vi "FPGA_ZAdjustment.vi"() -> ()   [LabVIEW 2014]
uses:
  <vilib>/rvi/Emulation/niFpgaGetClockAttributes.vi
  <vilib>/rvi/Emulation/niFpgaSctlEmulationGetInTimedLoop.vi
  <vilib>/rvi/Emulation/niFpgaEmulationReportErrorSimple.vi
  <vilib>/rvi/eio/common/nirviEmuTemplateMethod_errors.vi
  <vilib>/rvi/Emulation/niFpgaCriticalErrorInLSC.vi
  <vilib>/rvi/Emulation/niFpgaProcessEmulError.vi
  <vilib>/rvi/interface/RandomDataEmulation/niFpgaRandomDataHandleErrors.vi
  <vilib>/eio/EIONode/EIONode.xnode
  <vilib>/rvi/DataTransferAndStorage/Container/XNode/niFpgaContainer.xnode
  <vilib>/rvi/interface/RandomDataEmulation/nirviRandomDataFpgaReadWriteTemplate.vi
panel:
  out "Connector0/DIO0":bool
  out "Connector0/DIO1":bool
  out "Connector0/DIO2":bool
  out "ZRealTimePos":i16
  in  "stop":bool
  in  "ZOffset":i16
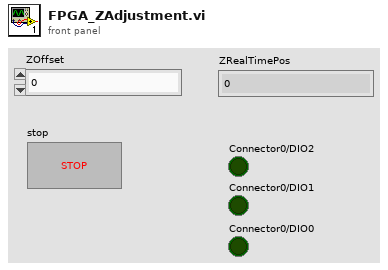
[diagram p1: front panel]
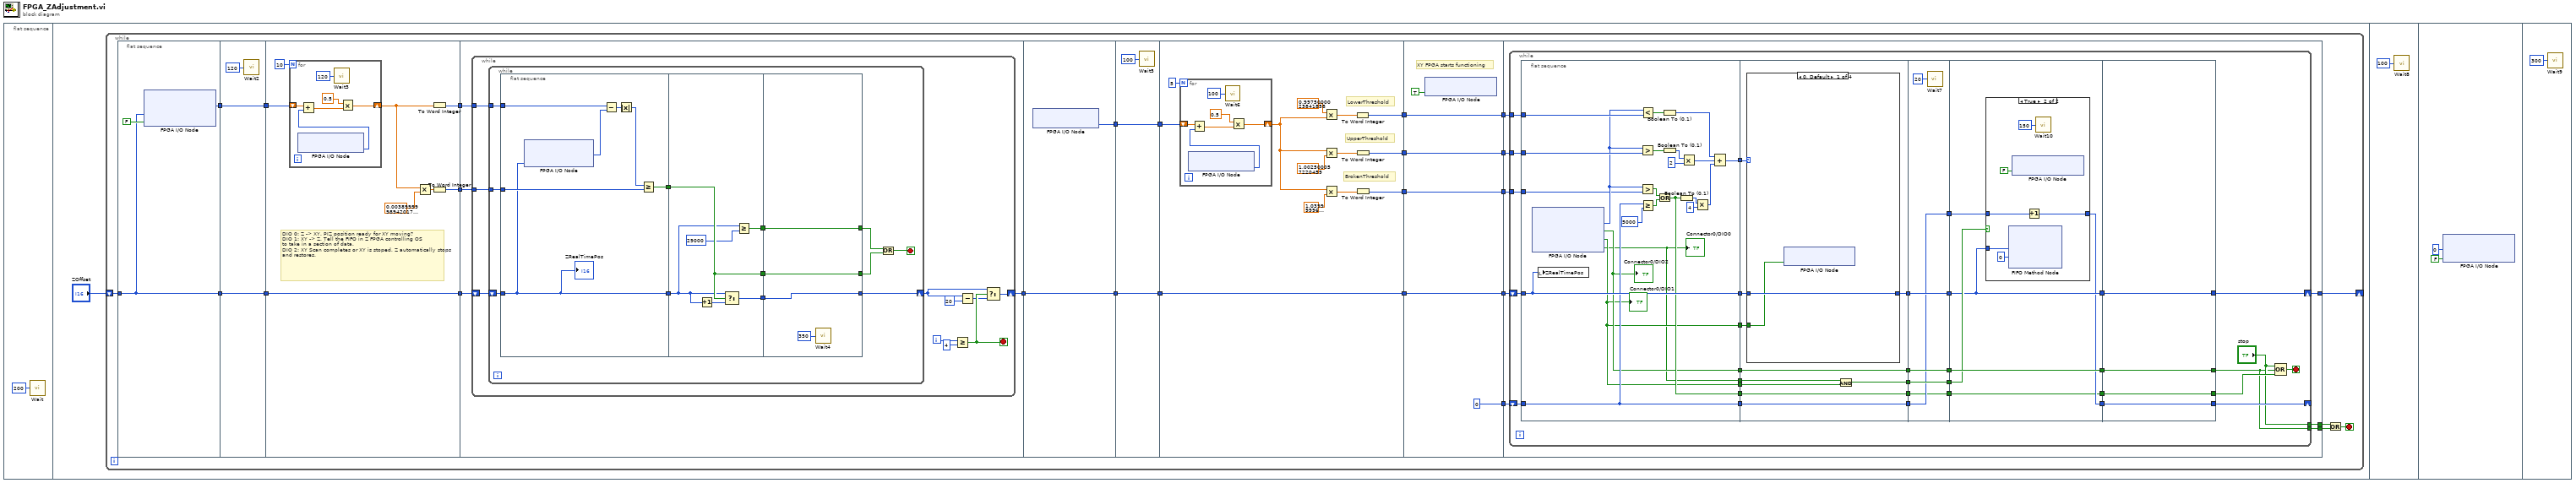
[diagram p0: block diagram]
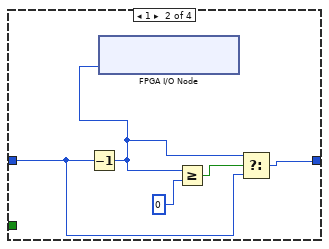
[diagram p2: hidden frame]
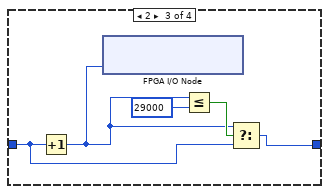
[diagram p3: hidden frame]
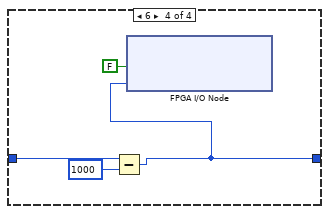
[diagram p4: hidden frame]
diagram:
  n1 = flat-sequence {
    frame #0 {
      n2 = call "Wait"("Count(uSec)"=u32 200) -> ()  [unwired: 1 out]
    }
    frame #1 {
      n3 = while {
        shift-right: [w7] -> _
        shift-left: "ZOffset" -> [w24]
        stop <- w5 stop-if-true
        n4 = flat-sequence {
          tunnel: [w31] -> w27
          tunnel: w24 -> [w29]
          tunnel: [w29] -> w22
          tunnel: [w33] -> w28
          tunnel: w27 -> [w33]
          tunnel: [w32] -> w23
          tunnel: w22 -> [w32]
          tunnel: w28 -> [w41]
          tunnel: [w37] -> w26
          tunnel: [w36] -> w25
          tunnel: w23 -> [w35]
          tunnel: [w35] -> w21
          tunnel: w26 -> [w52]
          tunnel: w25 -> [w51]
          tunnel: w21 -> [w50]
          tunnel: [w49] -> w20
          tunnel: w20 -> [w92]
          tunnel: [w93] -> w19
          tunnel: [w92] -> w10
          tunnel: w19 -> [w95]
          tunnel: [w95] -> w18
          tunnel: [w94] -> w11
          tunnel: w10 -> [w94]
          tunnel: w18 -> [w108]
          tunnel: [w100] -> w17
          tunnel: [w99] -> w15
          tunnel: [w98] -> w13
          tunnel: w11 -> [w97]
          tunnel: [w97] -> w8
          tunnel: w17 -> [w121]
          tunnel: [w121] -> w16
          tunnel: w15 -> [w120]
          tunnel: [w120] -> w14
          tunnel: w13 -> [w119]
          tunnel: [w119] -> w12
          tunnel: [w117] -> w9
          tunnel: w8 -> [w117]
          tunnel: [i16 0] -> w6
          tunnel: w16 -> [w129]
          tunnel: w14 -> [w128]
          tunnel: w12 -> [w127]
          tunnel: w9 -> [w126]
          tunnel: [w125] -> w7
          tunnel: w6 -> [w124]
          tunnel: [w123] -> w4
          tunnel: [w122] -> w3
          frame #0 {
            n5 = xnode "FPGA I/O Node"("Connector0/AO0"=w29, "Connector0/DIO0"=FALSE) -> ("Connector0/AI1"=w31:i16)  [unwired: 3 in, 3 out]
          }
          frame #1 {
            n6 = call "Wait2"("Count(uSec)"=u32 120) -> ()  [unwired: 1 out]
          }
          frame #2 {
            # "DIO 0: Z -> XY. PIZ position ready for XY moving?\nDIO 1: XY -> Z. Tell the FIFO in Z FPGA controlling OS\nto take in a section of data.\nDIO 2: XY Scan completes or XY is stoped, Z automatically stops and restores."
            n7 = for {
              N: 10 -> [_]
              shift-right: [w44] -> w39
              shift-left: w41 -> [w48]
              n8 = xnode "FPGA I/O Node"() -> ("Connector0/AI1"=w47:i16)  [unwired: 1 in, 1 out]
              n9 = Add(x=w48, y=w47) -> (x+y=w46:sgl)
              n10 = call "Wait3"("Count(uSec)"=u32 120) -> ()  [unwired: 1 out]
              n11 = Multiply(x=sgl 0.5, y=w46) -> (x*y=w44:sgl)
            }
            n12 = Multiply(x=w39, y=sgl 0.0039) -> (x*y=w38:sgl)
            n13 = To Word Integer(number=w39) -> (16bit integer=w37:i16)
            n14 = To Word Integer(number=w38) -> (16bit integer=w36:i16)
          }
          frame #3 {
            n15 = while {
              tunnel: w52 -> [w62]
              tunnel: w51 -> [w61]
              shift-right: [w58] -> w49
              shift-left: w50 -> [w60]
              i -> [w59]
              stop <- w57 stop-if-true
              n16 = while {
                tunnel: w62 -> [w74]
                tunnel: w61 -> [w73]
                shift-right: [w67] -> w56
                shift-left: w60 -> [w71]
                stop <- w65 stop-if-true
                n17 = flat-sequence {
                  tunnel: w74 -> [w81]
                  tunnel: w73 -> [w77]
                  tunnel: [w76] -> w72
                  tunnel: w71 -> [w75]
                  tunnel: [w75] -> w70
                  tunnel: w72 -> [w85]
                  tunnel: w70 -> [w84]
                  tunnel: [w86] -> w69
                  tunnel: [w85] -> w68
                  tunnel: [w82] -> w66
                  tunnel: w69 -> [w89]
                  tunnel: w68 -> [w90]
                  tunnel: [w90] -> w63
                  tunnel: [w89] -> w67
                  tunnel: [w88] -> w64
                  tunnel: w66 -> [w88]
                  frame #0 {
                    n18 = xnode "FPGA I/O Node"("Connector0/AO0"=w75) -> ("Connector0/AI1"=w80:i16)  [unwired: 2 in, 2 out]
                    n19 = Subtract(x=w81, y=w80) -> (x-y=w79:i16)
                    n20 = Absolute Value(x=w79) -> (abs(x)=w78:i16)
                    n21 = Greater Or Equal?(x=w78, y=w77) -> (x >= y?=w76:bool)
                    "ZRealTimePos" <- w75
                  }
                  frame #1 {
                    n22 = Increment(x=w84) -> (x+1=w87:i16)
                    n23 = Select(t=w84, s=w85, f=w87) -> (s? t:f=w86:i16)
                    n24 = Greater Or Equal?(x=w84, y=i16 29000) -> (x >= y?=w82:bool)
                  }
                  frame #2 {
                    n25 = call "Wait4"("Count(uSec)"=u32 350) -> ()  [unwired: 1 out]
                  }
                }
                n26 = Or(x=w64, y=w63) -> (x .or. y?=w65:bool)
              }
              n27 = Greater Or Equal?(x=w59, y=4) -> (x >= y?=w57:bool)
              n28 = Subtract(x=w56, y=i16 20) -> (x-y=w54:i16)
              n29 = Select(t=w56, s=w57, f=w54) -> (s? t:f=w58:i16)
            }
          }
          frame #4 {
            n30 = xnode "FPGA I/O Node"() -> ("Connector0/AI1"=w93:i16)  [unwired: 1 in, 1 out]
          }
          frame #5 {
            n31 = call "Wait5"("Count(uSec)"=u32 100) -> ()  [unwired: 1 out]
          }
          frame #6 {
            # "BrokenThreshold"
            # "UpperThreshold"
            # "LowerThreshold"
            n32 = for {
              N: 5 -> [_]
              shift-right: [w111] -> w101
              shift-left: w108 -> [w115]
              n33 = xnode "FPGA I/O Node"() -> ("Connector0/AI1"=w114:i16)  [unwired: 1 in, 1 out]
              n34 = Add(x=w115, y=w114) -> (x+y=w113:sgl)
              n35 = call "Wait6"("Count(uSec)"=u32 100) -> ()  [unwired: 1 out]
              n36 = Multiply(x=sgl 0.5, y=w113) -> (x*y=w111:sgl)
            }
            n37 = Multiply(x=sgl 0.9975 ("y"), y=w101) -> (x*y=w105:sgl)
            n38 = Multiply(x=w101, y=sgl 1.0025) -> (x*y=w104:sgl)
            n39 = Multiply(x=w101, y=sgl 1.04) -> (x*y=w102:sgl)
            n40 = To Word Integer(number=w105) -> (16bit integer=w100:i16)
            n41 = To Word Integer(number=w104) -> (16bit integer=w99:i16)
            n42 = To Word Integer(number=w102) -> (16bit integer=w98:i16)
          }
          frame #7 {
            # "XY FPGA starts functioning"
            n43 = xnode "FPGA I/O Node"("Connector0/DIO0"=TRUE) -> ()  [unwired: 1 in, 1 out]
          }
          frame #8 {
            n44 = while {
              tunnel: w129 -> [w162]
              tunnel: w128 -> [w161]
              tunnel: w127 -> [w160]
              shift-right: [w151] -> w125
              shift-left: w126 -> [w159]
              shift-right: [w143] -> _
              shift-left: w124 -> [w147]
              tunnel: ["stop"] -> w123
              tunnel: [w136] -> w122
              stop <- w139 stop-if-true
              n45 = flat-sequence {
                tunnel: w162 -> [w185]
                tunnel: w161 -> [w184]
                tunnel: w160 -> [w182]
                tunnel: w159 -> [w171]
                tunnel: [w172] -> w158
                tunnel: [w165] -> w157
                tunnel: [w171] -> w154
                tunnel: [w164] -> w150
                tunnel: w147 -> [w168]
                tunnel: [w168] -> w144
                tunnel: [w166] -> w142
                tunnel: [w164] -> w131
                tunnel: [w163] -> w130
                tunnel: w158 -> [w195]
                tunnel: w157 -> [w194]
                tunnel: [w194] -> w155
                tunnel: w154 -> [w193]
                tunnel: [w192] -> w153
                tunnel: w150 -> [w187]
                tunnel: [w188] -> w148
                tunnel: [w191] -> w145
                tunnel: w144 -> [w191]
                tunnel: w142 -> [w190]
                tunnel: [w190] -> w141
                tunnel: w131 -> [w189]
                tunnel: w130 -> [w186]
                tunnel: [w216] -> w156
                tunnel: w155 -> [w216]
                tunnel: w153 -> [w215]
                tunnel: [w215] -> w152
                tunnel: [w214] -> w149
                tunnel: w148 -> [w214]
                tunnel: [w213] -> w146
                tunnel: w145 -> [w213]
                tunnel: w141 -> [w212]
                tunnel: [w212] -> w140
                tunnel: w156 -> [w223]
                tunnel: w152 -> [w221]
                tunnel: w149 -> [w222]
                tunnel: w146 -> [w220]
                tunnel: w140 -> [w218]
                tunnel: [w223] -> w135
                tunnel: [w221] -> w134
                tunnel: [w219] -> w133
                tunnel: [w218] -> w132
                tunnel: [w231] -> w138
                tunnel: [w232] -> w143
                tunnel: [w233] -> w151
                tunnel: [w234] -> w136
                tunnel: w135 -> [w234]
                tunnel: w134 -> [w233]
                tunnel: w133 -> [w232]
                tunnel: w132 -> [w231]
                frame #0 {
                  n46 = xnode "FPGA I/O Node"() -> ("Connector0/AI1"=w183:i16, "Connector0/DIO2"=w165:bool, "Connector0/DIO1"=w164:bool, "Connector0/DIO0"=w163:bool)  [unwired: 4 in, 4 out]
                  "Connector0/DIO2" <- w165
                  "Connector0/DIO1" <- w164
                  "Connector0/DIO0" <- w163
                  n47 = local write "ZRealTimePos"(w171) -> ()
                  n48 = Greater?(x=w183, y=w184) -> (0:w180:bool)
                  n49 = Greater?(x=w183, y=w182) -> (0:w170:bool)
                  n50 = Less?(x=w183, y=w185) -> (x < y?=w181:bool)
                  n51 = Greater Or Equal?(x=w168, y=i16 5000) -> (x >= y?=w169:bool)
                  n52 = Or(x=w170, y=w169) -> (x .or. y?=w166:bool)
                  n53 = Boolean To (0,1)(Boolean=w180) -> (0, 1=w179:i16)
                  n54 = Boolean To (0,1)(Boolean=w181) -> (0, 1=w175:i16)
                  n55 = Boolean To (0,1)(Boolean=w166) -> (0, 1=w177:i16)
                  n56 = Multiply(x=w179, y=i16 2) -> (x*y=w174:i16)
                  n57 = Multiply(x=w177, y=i16 4) -> (x*y=w173:i16)
                  n58 = Compound Arithmetic op=ADD(w175, w174, w173) -> (w172:i16)
                }
                frame #1 {
                  n59 = case shown="0, Default" w195 {
                    tunnel: w193 -> [w197 w198 w203 w211]
                    tunnel: [w197 w200 w205 w209] -> w192
                    tunnel: w189 -> [w196 _ _ _]
                    frame 0, Default {
                      n60 = xnode "FPGA I/O Node"("Connector0/DIO0"=w196) -> ()  [unwired: 1 in, 1 out]
                    }
                    frame 1 {
                      n61 = Decrement(x=w198) -> (x-1=w199:i16)
                      n62 = xnode "FPGA I/O Node"("Connector0/AO0"=w199) -> ()  [unwired: 1 in, 1 out]
                      n63 = Greater Or Equal?(x=w199, y=i16 0) -> (x >= y?=w202:bool)
                      n64 = Select(t=w199, s=w202, f=w198) -> (s? t:f=w200:i16)
                    }
                    frame 2 {
                      n65 = Increment(x=w203) -> (x+1=w204:i16)
                      n66 = xnode "FPGA I/O Node"("Connector0/AO0"=w204) -> ()  [unwired: 1 in, 1 out]
                      n67 = Less Or Equal?(x=w204, y=i16 29000) -> (x <= y?=w206:bool)
                      n68 = Select(t=w204, s=w206, f=w203) -> (s? t:f=w205:i16)
                    }
                    frame 6 {
                      n69 = Subtract(x=w211, y=i16 1000) -> (x-y=w209:i16)
                      n70 = xnode "FPGA I/O Node"("Connector0/DIO0"=FALSE, "Connector0/AO0"=w209) -> ()  [unwired: 2 in, 2 out]
                    }
                  }
                  n71 = And(x=w186, y=w187) -> (x .and. y?=w188:bool)
                }
                frame #2 {
                  n72 = call "Wait7"("Count(uSec)"=u32 20) -> ()  [unwired: 1 out]
                }
                frame #3 {
                  n73 = case shown="True" w222 {
                    tunnel: w221 -> [_ w229]
                    tunnel: w220 -> [w224 w228]
                    tunnel: [w224 w227] -> w219
                    frame False {
                    }
                    frame True {
                      n74 = xnode ("FIFO Method Node")("Element"=w229, "Timeout"=0) -> ()  [unwired: 1 in, 2 out]
                      n75 = xnode "FPGA I/O Node"("Connector0/DIO0"=FALSE) -> ()  [unwired: 1 in, 1 out]
                      n76 = Increment(x=w228) -> (x+1=w227:i16)
                      n77 = call "Wait10"("Count(uSec)"=u32 150) -> ()  [unwired: 1 out]
                    }
                  }
                }
                frame #4 {
                }
              }
              n78 = Compound Arithmetic op=OR("stop", w136, w138) -> (w139:bool)
            }
          }
        }
        n79 = Or(x=w4, y=w3) -> (x .or. y?=w5:bool)
      }
    }
    frame #2 {
      n80 = call "Wait8"("Count(uSec)"=u32 100) -> ()  [unwired: 1 out]
    }
    frame #3 {
      n81 = xnode "FPGA I/O Node"("Connector0/AO0"=i16 0, "Connector0/DIO0"=FALSE) -> ()  [unwired: 2 in, 2 out]
    }
    frame #4 {
      n82 = call "Wait9"("Count(uSec)"=u32 300) -> ()  [unwired: 1 out]
    }
  }
